vi "SetVelocityTank.vi"(8 "error in (no error)":errorcluster, 9 "rightVelocitySetpointInput":dbl, 10 "leftVelocitySetpointInput":dbl) -> (0 "error out":errorcluster)   [LabVIEW 2016, in "DriveBase.lvclass"]
uses:
  DriveBase.lvclass
  DriveBase.lvclass/DriveBase.ctl
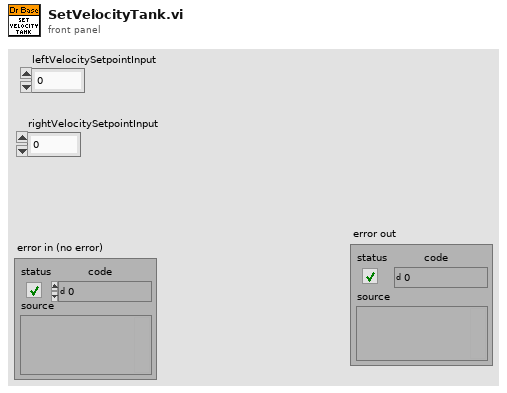
[diagram p1: front panel]
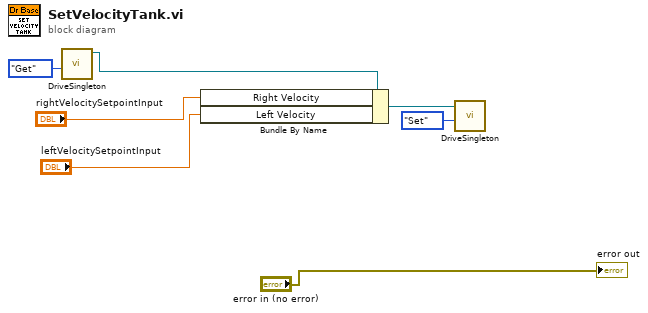
[diagram p0: block diagram]
diagram:
  n1 = call "DriveSingleton.vi"("Get/Set"=enum16{"Get", "Set"}."Get") -> ("DriveBase.lvclass 2"=w5:refnum<class "DriveBase.lvclass">)  [unwired: 9 in, 1 out]
  n2 = Bundle By Name(cluster=w5, "Right Velocity"="rightVelocitySetpointInput", "Left Velocity"="leftVelocitySetpointInput") -> (w2:refnum<class "DriveBase.lvclass">)
  n3 = call "DriveSingleton.vi"("Get/Set"=enum16{"Get", "Set"}."Set", "DriveBase.lvclass"=w2) -> ()  [unwired: 8 in, 2 out]
  "error out" <- "error in (no error)"
